vi "HealthAndStatus.vi"(11 "HealthAndStatusSettings":T1={"InternalHealthAndStatusFIFO"="InternalHealthAndStatusFIFO", "HealthAndStatusQueryFIFO"="HealthAndStatusQueryFIFO", "HealthAndStatusResponseFIFO"="HealthAndStatusResponseFIFO", "HealthAndStatusMemory"="HealthAndStatusMemory", "MemorySize"=0}) -> ()   [LabVIEW 2018, in "FPGAHealthAndStatus.lvlib"]
uses:
  FPGAHealthAndStatus.lvlib
  DataTypes/HealthAndStatusSettings.ctl
  <vilib>/rvi/DataTransferAndStorage/Container/Common/niFpgaContainerExecOnDevCompGetState.vi
  <vilib>/rvi/Emulation/niFpgaEmulationIsFPGAContextNoSignature.vi
  <vilib>/rvi/Emulation/niFpgaSctlEmulationGetInTimedLoop.vi
  <vilib>/rvi/errors/niFpgaSetErrorForExecOnDevCompSimple.vi
  <vilib>/rvi/eio/common/nirviEmuReportErrorAndStop.vi
  <vilib>/rvi/DataTransferAndStorage/Container/Common/niFpgaContainerGetUniqueNameForEmu.vi
  <vilib>/rvi/FIFO/Fifo_Resource/nirvififoEmulationSetSize.vi
  <vilib>/rvi/FIFO/Fifo_Resource/nirviFifoEmulationQueueMgr.vi
  <instcachedir>/0/nirviFifoEmulationQueueMgr_E5CAEC123FF24DC58D834DCA3CDAA9B5.lvgen/nirviFifoEmulationQueueMgr_E5CAEC123FF24DC58D834DCA3CDAA9B5_003.vi
  <vilib>/rvi/FIFO/Fifo_Resource/nirvififoEmulationDetermineInputValidOut.vi
  <vilib>/rvi/FIFO/Fifo_Resource/nirvififoEmulationCreateLock.vi
  <vilib>/rvi/Emulation/niFpgaProcessEmulError.vi
  <vilib>/rvi/FIFO/Fifo_Resource/nirvififoEmulationObtainLock.vi
  <vilib>/rvi/FIFO/Fifo_Resource/nirvififoEmulationReleaseLock.vi
  <vilib>/rvi/occurrence/nirviWaitOnOccurrenceBase.vi
  <vilib>/rvi/errors/nirviReportUnexpectedCaseInternalError.vi
  <vilib>/rvi/errors/nirviReportUnexpectedCaseInternalError (U32).vi
  <vilib>/Utility/error.llb/Clear Errors.vi
  <vilib>/rvi/interface/RandomDataEmulation/niFpgaRandomDataHandleErrors.vi
  <vilib>/rvi/DataTransferAndStorage/Container/XNode/niFpgaContainer.xnode
  <vilib>/rvi/FIFO/Fifo_Resource/niFpgaFifoEmulationRefIn.vi
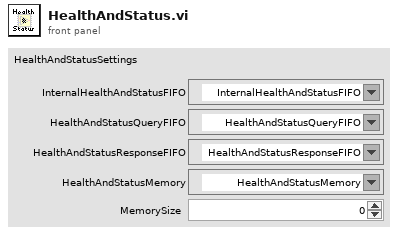
[diagram p1: front panel]
types:
  T1 = typedef "FPGAHealthAndStatus.lvlib/HealthAndStatusSettings.ctl" = cluster{"InternalHealthAndStatusFIFO":refnum<k21>, "HealthAndStatusQueryFIFO":refnum<k21>, "HealthAndStatusResponseFIFO":refnum<k21>, "HealthAndStatusMemory":refnum<k21>, "MemorySize":i32}
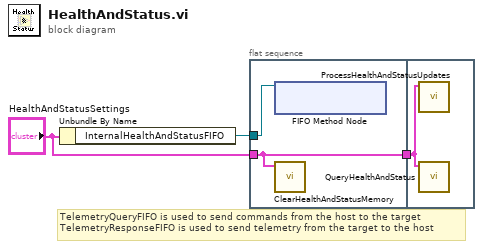
[diagram p0: block diagram]
diagram:
  # "TelemetryQueryFIFO is used to send commands from the host to the target\nTelemetryResponseFIFO is used to send telemetry from the target to the host"
  n1 = Unbundle By Name("HealthAndStatusSettings") -> ("InternalHealthAndStatusFIFO"=w2:refnum<k21>)
  n2 = flat-sequence {
    tunnel: [w4] -> w3
    tunnel: w2 -> [w5]
    tunnel: "HealthAndStatusSettings" -> [w4]
    tunnel: w3 -> [w6]
    frame #0 {
      n3 = xnode ("FIFO Method Node")("FIFO In"=w5) -> ()  [unwired: 1 out]
      n4 = call "ClearHealthAndStatusMemory.vi"("HealthAndStatusSettings"=w4) -> ()  [unwired: 11 in]
    }
    frame #1 {
      n5 = call "ProcessHealthAndStatusUpdates.vi"("HealthAndStatusSettings"=w6) -> ()  [unwired: 11 in]
      n6 = call "QueryHealthAndStatus.vi"("HealthAndStatusSettings"=w6) -> ()  [unwired: 11 in]
    }
  }
